vi "RichToFlatcif_manager_DestroyResponse.vi"(5 "OutputClusterType":T1, 11 "InputCluster":T2) -> (3 "OutputCluster":T1)   [LabVIEW 2021, in "CIF_Manager_server.lvlib"]
uses:
  CIF_Manager_server.lvlib
  cif_manager_DestroyResponse.ctl
  cif_manager_DestroyResponse_Flat.ctl
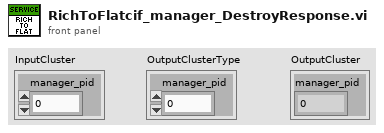
[diagram p1: front panel]
types:
  T1 = typedef "CIF_Manager_server.lvlib/cif_manager_DestroyResponse_Flat.ctl" = cluster{"manager_pid":u32}
  T2 = typedef "CIF_Manager_server.lvlib/cif_manager_DestroyResponse.ctl" = cluster{"manager_pid":u32}
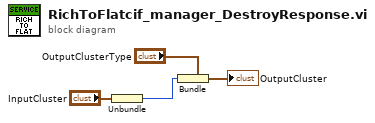
[diagram p0: block diagram]
diagram:
  n1 = Unbundle "Unbundle"("InputCluster") -> ("manager_pid"=w1:u32)
  n2 = Bundle "Bundle"(cluster="OutputClusterType", "manager_pid"=w1) -> (→"OutputCluster":T1)
